vi "Read InfoCCDmode.vi"(8 "error in (no error)":errorcluster, 11 "S4GUI in":refnum<class "S4GUI.lvclass">) -> (0 "error out":errorcluster, 2 "InfoCCDmode":T1 caption="INFORMATION OF SELECTED MODE", 3 "S4GUI out":refnum<class "S4GUI.lvclass">)   [LabVIEW 2018, in "S4GUI.lvclass"]
uses:
  S4GUI.lvclass
  S4GUI.lvclass/S4GUI.ctl
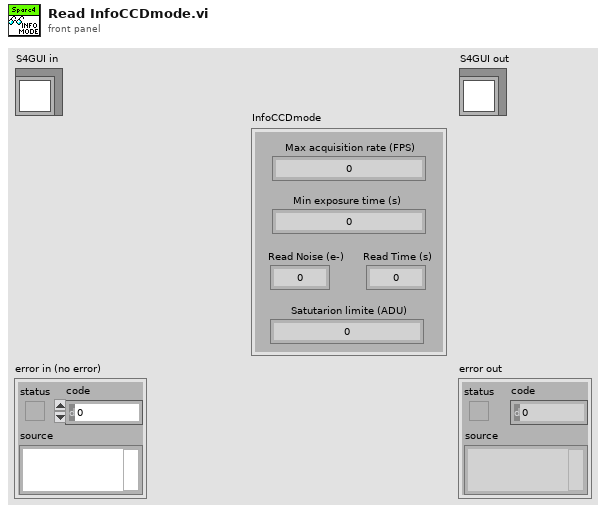
[diagram p1: front panel]
types:
  T1 = cluster{"AcqRate":dbl, "MinExpTime":dbl, "readNoise":dbl, "readTime":dbl, "SatLim":dbl}
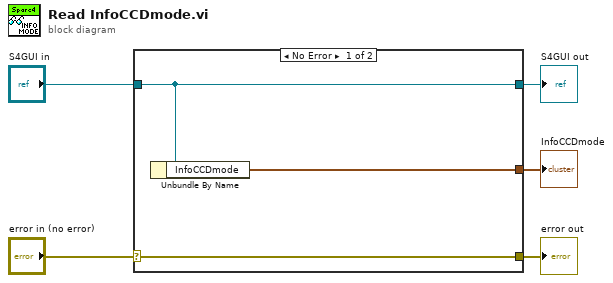
[diagram p0: block diagram]
diagram:
  n1 = case shown="No Error" "error in (no error)" {
    selector: "error in (no error)" -> [w8 w9]
    tunnel: [w8 w9] -> w4
    tunnel: [w7 w10] -> w2
    tunnel: "S4GUI in" -> [w7 w10]
    tunnel: [w6 _] -> w1
    frame No Error {
      n2 = Unbundle By Name(w7) -> ("InfoCCDmode"=w6:T1)
    }
    frame Error {
    }
  }
  "error out" <- w4
  "S4GUI out" <- w2
  "InfoCCDmode" <- w1
